vi "XIPIN_802.16e_CTC_Encoder_3_0.vi"   [LabVIEW 2017]
doc: "The Xilinx 802.16e Convolutional Turbo Coder LogiCORE is a drop-in module for Virtex-4(TM), Virtex-5(TM), Virtex-6(TM), Spartan-3(TM) and Spartan-6(TM) families of FPGA. It is a high-speed, compact module for generating coded data streams according to the IEEE Std 802.16e-2005 and IEEE Std 802.16-2004/Cor1-2005 standard, OFDMA PHY layer. (Section 8.4.9.2.3) The core is fully synchronous, using a single clock, and integrates seamlessly with the Xilinx design flow.\n------------------------------------\n<b>Need License</b> : Yes"
uses:
  <vilib>/rvi/XilinxIP/XIPIN_XNode/niFpgaXIPIN.xnode
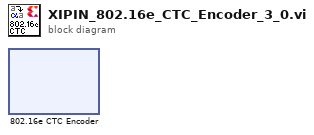
[diagram p0: block diagram]
diagram:
  n1 = xnode ("802.16e CTC Encoder")() -> ()
